vi "Query Marker.vi"(8 "error in (no error)":errorcluster, 10 "Marker Number (1)":u32=1 min=1, 11 "SA-ESA in":refnum<class "SA-ESA.lvclass">) -> (0 "error out":errorcluster, 1 "Marker Level":dbl, 2 "Marker Frequency/Time":dbl, 3 "SA-ESA out":refnum<class "SA-ESA.lvclass">)   [LabVIEW 2020, in "SA-ESA.lvclass"]
uses:
  SA-ESA.lvclass
  C:/Sandbox/RF Bench/Source Code/WiSpry Test Framework/Instruments/Instrument.lvclass
  Instrument.lvclass/Instrument.ctl
  Instrument.lvclass
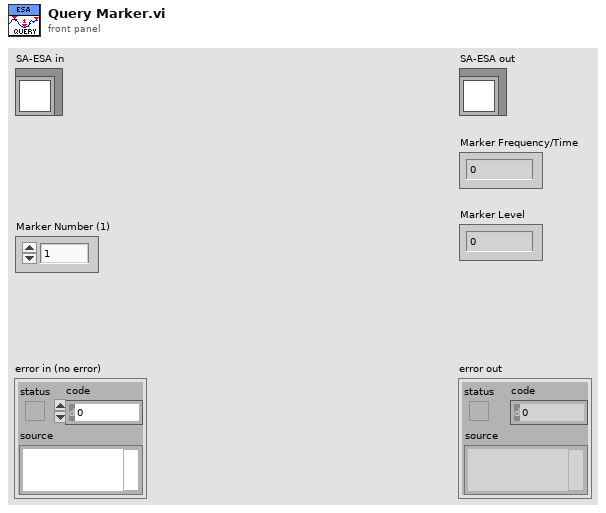
[diagram p1: front panel]
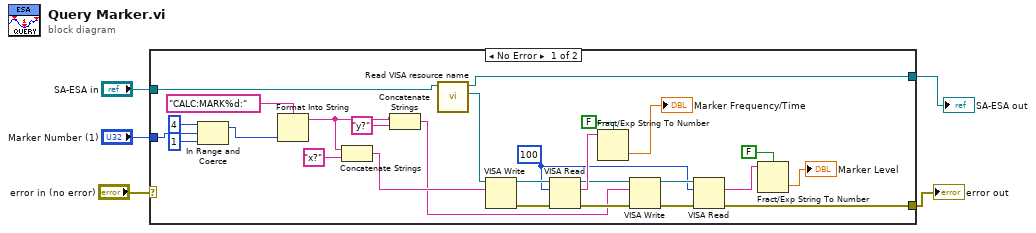
[diagram p0: block diagram]
diagram:
  n1 = case shown="No Error" "error in (no error)" {
    selector: "error in (no error)" -> [_ w33]
    tunnel: "SA-ESA in" -> [w24 w34]
    tunnel: "Marker Number (1)" -> [w32 _]
    tunnel: [w7 w33] -> w2
    tunnel: [w6 w34] -> w1
    frame No Error {
      w11 = u32 100 ("byte count")
      n2 = In Range and Coerce(upper limit=u32 4, x=w32, lower limit=u32 1) -> (coerced(x)=w28:u32)  [unwired: 1 out]
      n3 = Format Into String(format string="CALC:MARK%d:", w28) -> (resulting string=w26:string)  [unwired: 2 in, 1 out]
      n4 = Concatenate Strings(w26, "x?" ("string")) -> (w22:string)
      n5 = Concatenate Strings(w26, "y?" ("string")) -> (w12:string)
      n6 = call "Read VISA resource name.vi"("Instrument in"=w24) -> ("VISA resource name"=w23:refnum<visa-resource-name>, "Instrument out"=w6:refnum<class "SA-ESA.lvclass">)  [unwired: 9 in]
      n7 = VISA Write(VISA resource name=w23, write buffer=w22) -> (VISA resource name out=w20:refnum<visa-resource-name>, error out=w21:errorcluster)  [unwired: 1 in, 1 out]
      n8 = VISA Read(VISA resource name=w20, byte count=w11, error in (no error)=w21) -> (VISA resource name out=w14:refnum<visa-resource-name>, read buffer=w19:string, error out=w13:errorcluster)  [unwired: 1 out]
      n9 = Fract/Exp String To Number(use system decimal point (T)=FALSE, string=w19) -> (number=→"Marker Frequency/Time":dbl)  [unwired: 2 in, 1 out]
      n10 = VISA Write(VISA resource name=w14, write buffer=w12, error in (no error)=w13) -> (VISA resource name out=w16:refnum<visa-resource-name>, error out=w15:errorcluster)  [unwired: 1 out]
      n11 = VISA Read(VISA resource name=w16, byte count=w11, error in (no error)=w15) -> (read buffer=w9:string, error out=w7:errorcluster)  [unwired: 2 out]
      n12 = Fract/Exp String To Number(use system decimal point (T)=FALSE, string=w9) -> (number=→"Marker Level":dbl)  [unwired: 2 in, 1 out]
    }
    frame Error {
    }
  }
  "error out" <- w2
  "SA-ESA out" <- w1
